vi "McPherson Setup for new units.vi"(6 "Cluster":T1 {"Duration" format="%.2f"; "End" format="%.2f"; "Begin" format="%.2f"; "GOTO" format="%.2f"}, 9 "Old Cluster":T1 {"Duration" format="%.2f"; "End" format="%.2f"; "Begin" format="%.2f"; "GOTO" format="%.2f"}) -> (0 "ClusterOutput":T1 {"Duration" format="%.2f"; "End" format="%.2f"; "Begin" format="%.2f"; "GOTO" format="%.2f"}, 1 "Display":T3 {"Range"."Increment" format="%.2f"; "Range"."Maximum" format="%.2f"; "Range"."Minimum" format="%.2f"}, 2 "Speed Output":i16, 3 "Setpoint":T2, 4 "EndStep":i32, 5 "BeginStep":i32)   [LabVIEW 2024]
uses:
  File and save/X-Axis Converter.llb/X-Axis Converter.vi
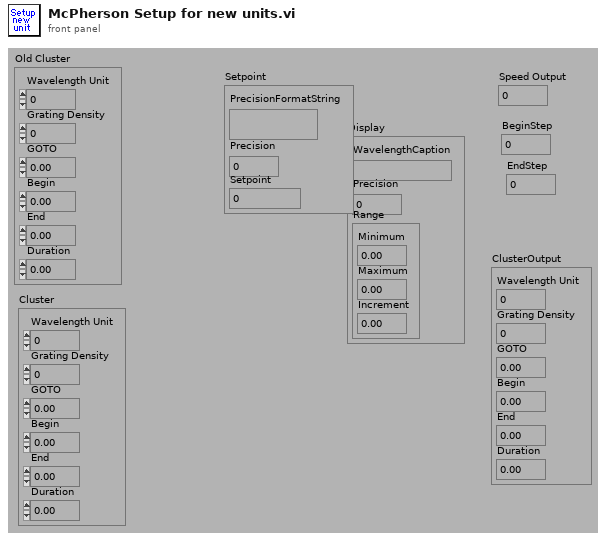
[diagram p1: front panel]
types:
  T1 = cluster{"Wavelength Unit":u8, "Grating Density":u8, "GOTO":dbl, "Begin":dbl, "End":dbl, "Duration":dbl}
  T2 = cluster{"PrecisionFormatString":string, "Precision":u8, "Setpoint":i32}
  T3 = cluster{"WavelengthCaption":string, "Precision":u8, "Range":cluster{"Minimum":dbl, "Maximum":dbl, "Increment":dbl}}
  T4 = cluster{"Wavelength Unit":u8, "Grating Density":u8, "Central WL output":dbl, "Central WL output":dbl, "Central WL output":dbl, "Duration":dbl}
  T5 = cluster{"X-Axis Unit String":string, "Precision":i32, cluster{dbl, dbl, dbl}}
  T6 = cluster{"UnitFormatString":string, "Precision":i32, "Stepper Position Output":i32}
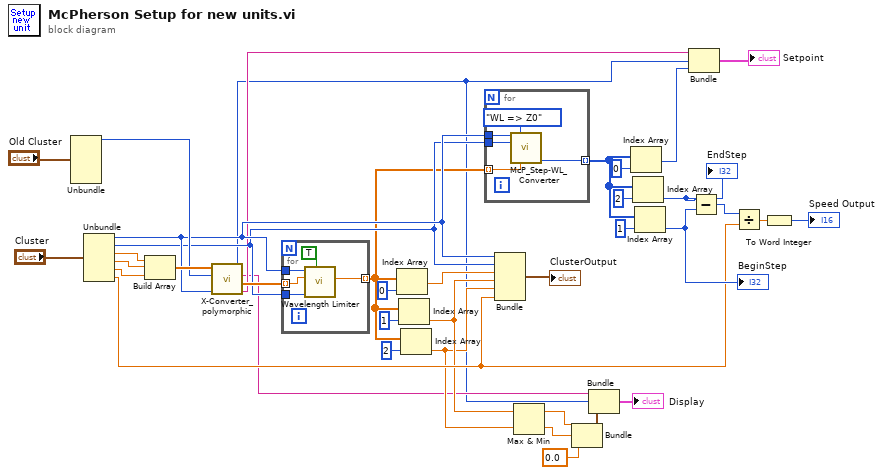
[diagram p0: block diagram]
diagram:
  n1 = Unbundle("Old Cluster") -> ("Wavelength Unit"=w28:u8)  [unwired: 5 out]
  n2 = Unbundle("Cluster") -> ("Wavelength Unit"=w22:u8, "Grating Density"=w21:u8, "GOTO"=w35:dbl, "Begin"=w34:dbl, "End"=w33:dbl, "Duration"=w12:dbl)
  n3 = Build Array(w35, w34, w33) -> (w30:dbl[])
  n4 = call-poly "X-Converter_polymorphic.vi"("X-Axis Unit"=w22, "Old X-Axis Unit"=w28, "X-Axis input"=w30) -> ("UnitFormatString"=w8:string, "X-Axis Output"=w29:dbl[], "X-Axis Unit String"=w3:string, "Precision"=w1:i32)  [unwired: 2 in]
  n5 = for {
    tunnel: w29 -> [w43] mode=indexing
    tunnel: w22 -> [w42]
    tunnel: w21 -> [w41]
    tunnel: [w40] -> w20 mode=indexing
    n6 = call "Wavelength Limiter.vi"("Range Limiter(F) or WL limiter"=TRUE, "Current Grating Density"=w41, "Central WL Input"=w43, "X-Axis"=w42) -> ("Central WL output"=w40:dbl)  [unwired: 1 in, 3 out]
  }
  n7 = Index Array(array=w20, index=0 ("Index")) -> (element=w24:dbl)
  n8 = Index Array(array=w20, index=1 ("Index")) -> (element=w7:dbl)
  n9 = Index Array(array=w20, index=2 ("Index")) -> (element=w6:dbl)
  n10 = for {
    tunnel: w22 -> [w48]
    tunnel: w21 -> [w47]
    tunnel: w20 -> [w46] mode=indexing
    tunnel: [w45] -> w16 mode=indexing
    n11 = call "McP_Step-WL_Converter.vi"("Wavelength Unit"=w48, "Option (Z0 <=> WL)"=enum16{"Z0 => WL", "WL => Z0", "Update WL only"}."WL => Z0", "Grating Density"=w47, "Wavelength Input"=w46) -> ("Stepper Position Output"=w45:i32)  [unwired: 4 in, 7 out]
  }
  n12 = Bundle("Wavelength Unit"=w22, "Grating Density"=w21, "Central WL output"=w24, "Central WL output"=w7, "Central WL output"=w6, "Duration"=w12) -> (→"ClusterOutput":T4)  [unwired: 1 in]
  n13 = Max & Min(x=w7, y=w6) -> (max(x,y)=w5:dbl, min(x,y)=w4:dbl)
  n14 = Bundle(w5, w4, 0.0) -> (w37:cluster{dbl, dbl, dbl})  [unwired: 1 in]
  n15 = Bundle("X-Axis Unit String"=w3, "Precision"=w1, w37) -> (→"Display":T5)  [unwired: 1 in]
  n16 = Index Array(array=w16, index=0 ("Index")) -> (element=w10:i32)
  n17 = Index Array(array=w16, index=2 ("Index")) -> (element=w15:i32)
  "EndStep" <- w15
  n18 = Index Array(array=w16, index=1 ("Index")) -> (element=w14:i32)
  "BeginStep" <- w14
  n19 = Bundle("UnitFormatString"=w8, "Precision"=w1, "Stepper Position Output"=w10) -> (→"Setpoint":T6)  [unwired: 1 in]
  n20 = Subtract(x=w15, y=w14) -> (x-y=w13:i32)
  n21 = Divide(x=w13, y=w12) -> (x/y=w11:dbl)
  n22 = To Word Integer(number=w11) -> (16bit integer=→"Speed Output":i16)
